vi "xmlNodecreate.vi"(1 "SN":string, 2 "TestResult":bool, 3 "path":path caption="路径", 4 "error in (no error)":errorcluster caption="错误输入（无错误）") -> (0 "error out":errorcluster)   [LabVIEW 2011]
uses:
  D:/2. HPTS_VNA_Rev2.7.1.0/Data/xmlFunction.dll
  Data/xmlFunction.dll
  <vilib>/xml/Load XML File.vi
  <vilib>/xml/Close Reference(Node).vi
  <vilib>/xml/NI_XML.lvlib
  program files/worksoftware/Labview/resource/objmgr/DOMUserDefRef.rc
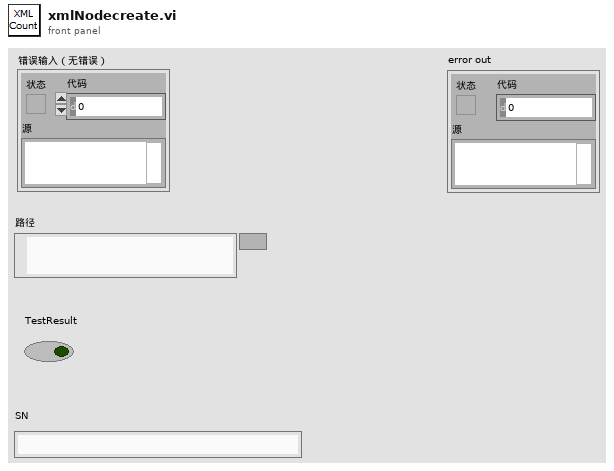
[diagram p1: front panel]
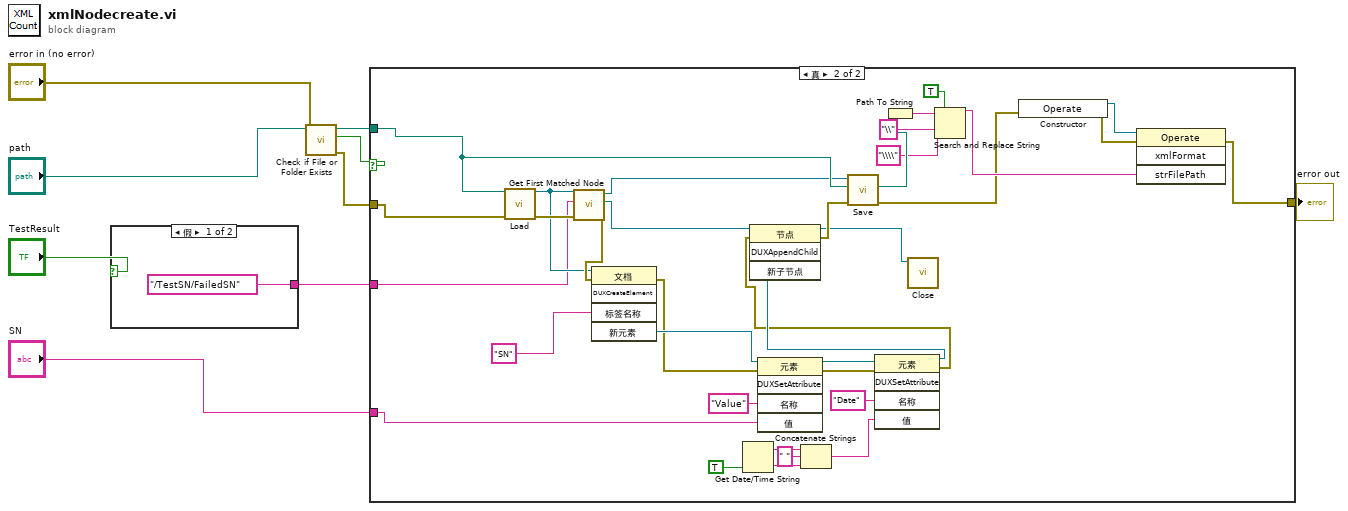
[diagram p0: block diagram]
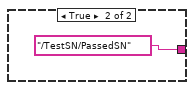
[diagram p2: hidden frame]
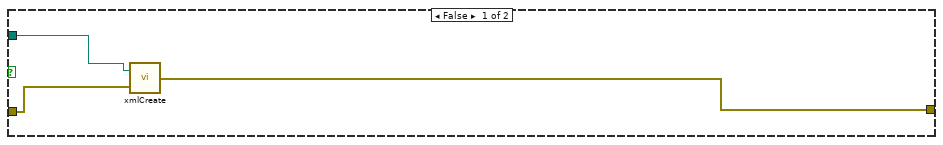
[diagram p3: hidden frame]
diagram:
  n1 = case shown="假" "TestResult" {
    tunnel: ["/TestSN/FailedSN" "/TestSN/PassedSN"] -> w5
    frame False {
    }
    frame True {
    }
  }
  n2 = call <vilib>:"Check if File or Folder Exists.vi"("error in (no error)"="error in (no error)", "path"="path") -> ("error out"=w3:errorcluster, "file or folder exists?"=w8:bool, "dup path"=w7:path)  [unwired: 7 in]
  n3 = case shown="真" w8 {
    tunnel: w7 -> [w14 w49]
    tunnel: w5 -> [_ w39]
    tunnel: "SN" -> [_ w29]
    tunnel: w3 -> [w12 w25]
    tunnel: [w13 w15] -> w1
    frame False {
      n4 = call "xmlCreate.vi"("error in (no error)"=w12, "XML file path"=w14) -> ("error out"=w13:errorcluster)
    }
    frame True {
      n5 = call-poly <vilib>:"Load.vi"("path to XML document"=w49, "error in (no error)"=w25) -> ("DOM document out"=w44:refnum<k20>, "error out"=w47:errorcluster)  [unwired: 11 in, 1 out]
      n6 = call <vilib>:"Get First Matched Node.vi"("error in (no error)"=w47, "XPath expression"=w39, "node in"=w44) -> ("error out"=w46:errorcluster, "node result"=w45:refnum<k20>, "node out"=w40:refnum<k20>)  [unwired: 6 in]
      n7 = invoke class="文档" method="DUXCreateElement"(reference=w44, error in=w46, "标签名称"="SN") -> (error out=w28:errorcluster, "新元素"=w42:refnum<k20>)  [unwired: 2 in, 3 out]
      n8 = Get Date/Time String(want seconds? (F)=TRUE) -> (date string=w32:string, time string=w31:string)  [unwired: 2 out]
      n9 = invoke class="元素" method="DUXSetAttribute"(reference=w42, error in=w28, "名称"="Value", "值"=w29) -> (reference out=w37:refnum<k20>, error out=w27:errorcluster)  [unwired: 1 in, 3 out]
      n10 = Concatenate Strings(w32, " " ("string"), w31) -> (w30:string)
      n11 = invoke class="元素" method="DUXSetAttribute"(reference=w37, error in=w27, "名称"="Date", "值"=w30) -> (reference out=w36:refnum<k20>, error out=w26:errorcluster)  [unwired: 1 in, 3 out]
      n12 = invoke class="节点" method="DUXAppendChild"(reference=w45, error in=w26, "新子节点"=w36) -> (reference out=w41:refnum<k20>, error out=w43:errorcluster)  [unwired: 1 in, 2 out]
      n13 = call <vilib>:"Save.vi"("error in (no error)"=w43, "XML file path"=w49, "DOM document in"=w40) -> ("error out"=w17:errorcluster, "XML file path out"=w24:path)  [unwired: 6 in, 1 out]
      n14 = Path To String(path=w24) -> (string=w23:string)
      n15 = call-poly <vilib>:"Close.vi"("node"=w41) -> ()  [unwired: 1 in, 8 out]
      n16 = Search and Replace String(replace all?=TRUE ("替换全部？(F)"), input string=w23, search string="\\" ("搜索字符串"), replace string="\\\\" ("替换字符串(\"\")")) -> (result string=w18:string)  [unwired: 4 in, 3 out]
      n17 = constructor class="Operate"(error in=w17) -> (reference out=w19:refnum<k24>, error out=w16:errorcluster)  [unwired: 2 in, 1 out]
      n18 = invoke class="Operate" method="xmlFormat"(reference=w19, error in=w16, "strFilePath"=w18) -> (error out=w15:errorcluster)  [unwired: 1 in, 3 out]
    }
  }
  "error out" <- w1
